vi "Read Measurement 2 Channels.vi"(6 "Measurement Type (0: Phase)":i32(ring) items=["Phase", "Delay", "DelayRR", "DelayRF", "DelayFR", "DelayFF"], 8 "error in (no error)":errorcluster, 9 "Channel 2 (2: Channel 2)":i32(ring)=2 items=["Channel 1"=1, "Channel 2"=2, "Channel 3"=3, "Channel 4"=4], 10 "Channel 1 (1: Channel 1)":i32(ring)=1 items=["Channel 1"=1, "Channel 2"=2, "Channel 3"=3, "Channel 4"=4], 11 "Tektronic in":refnum<class "Tektronic.lvclass">) -> (0 "error out":errorcluster, 1 "Measurement":dbl, 2 "Units":string, 3 "Tektronic out":refnum<class "Tektronic.lvclass">)   [LabVIEW 2020, in "Controlador.lvlib" / "Tektronic.lvclass"]
uses:
  Tektronic.lvclass
  C:/Users/scrap/Fork/Modulo_Cloneable_DQMH/Libraries/Controlador/Class/Osciloscope/Osciloscope.lvclass
  Osciloscope/Osciloscope.lvclass/Osciloscope.ctl
  Osciloscope/Read COM.vi
  <instrlib>/Tektronix TDS 200 1000 2000 Series/Tektronix TDS 200 1000 2000 Series.lvlib
  Osciloscope/Osciloscope.lvclass
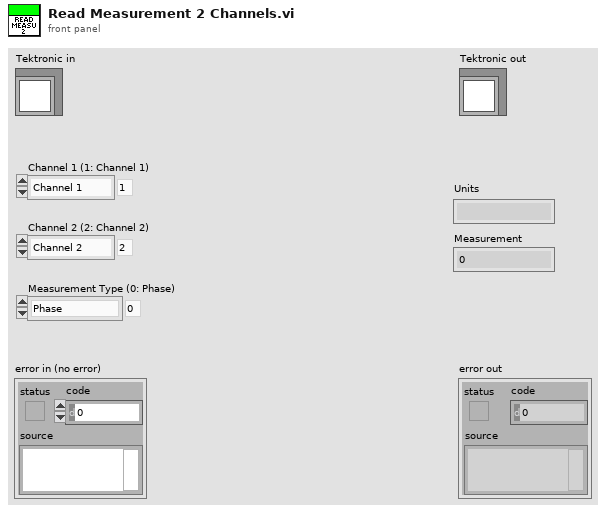
[diagram p1: front panel]
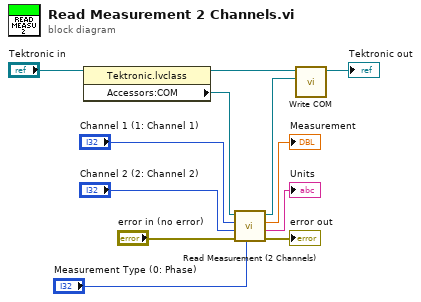
[diagram p0: block diagram]
diagram:
  n1 = property class="Tektronic.lvclass"(reference="Tektronic in") -> (reference out=w2:refnum<class "Tektronic.lvclass">, "Accessors:COM"=w5:refnum<visa-resource-name>)  [unwired: 1 in, 1 out]
  n2 = call <instrlib>:"Read Measurement (2 Channels).vi"("Measurement Type (0: Phase)"="Measurement Type (0: Phase)", "error in (no error)"="error in (no error)", "Channel 2 (2: Channel 2)"="Channel 2 (2: Channel 2)", "Channel 1 (1: Channel 1)"="Channel 1 (1: Channel 1)", "VISA resource name"=w5) -> ("error out"=→"error out":errorcluster, "Units"=→"Units":string, "Measurement"=→"Measurement":dbl, "VISA resource name out"=w3:refnum<visa-resource-name>)  [unwired: 3 in]
  n3 = call "Write COM.vi"("COM"=w3, "Osciloscope in"=w2) -> ("Osciloscope out"=→"Tektronic out":refnum<class "Tektronic.lvclass">)  [unwired: 8 in, 1 out]
